vi "TonePattern-Initialize.vi"(0 "Tone Cloud":T2={"Freq"={"Min (Hz)"=500.0, "Max (Hz)"=8000.0, "#/octave"=4}, "Time"={"Duration (ms)"=50.0, "Interval (ms)"=50.0, "Ramp (ms)"=5.0}, "Pattern"={"# rand"=2.0, "reg fraction"=1.0, "Rcyc"=1, "pattern"=enum."REG", "Lsignal (cyc)"={"Min"=0, "Max"=0}, "Trans (cyc)"={"Min"=0, "Max"=0}}} caption="ToneCloud", 7 "Sampling rate (Hz)":dbl=50000.0, 9 "Npts":i32, 11 "error in (no error)":errorcluster) -> (3 "#frames":i32, 4 "Freqs":dbl[](array[numeric]), 8 "Data":T1={"Tones"=array2x2500[5000 elements], "Mask"=[1], "Index"=0, "pts/clock"=2500, "leftover"=0, "pts/tone"=0, "transition"=0, "nrepeat"=0}, 15 "error out":errorcluster)   [LabVIEW 2020]
uses:
  TonePattern-Properties.ctl
  TonePattern-Data.ctl
  TonePattern-Initialization Action.ctl
  Utility VIs/Math VIs/LinSpace (x0-dx-npts).vi
  Utility VIs/Array Manipulation VIs/Irregular Array Subset (I32).vi
  <vilib>/Analysis/1siggen.llb/Riffle Array (I32).vi
  <vilib>/Analysis/NI_AALBase.lvlib
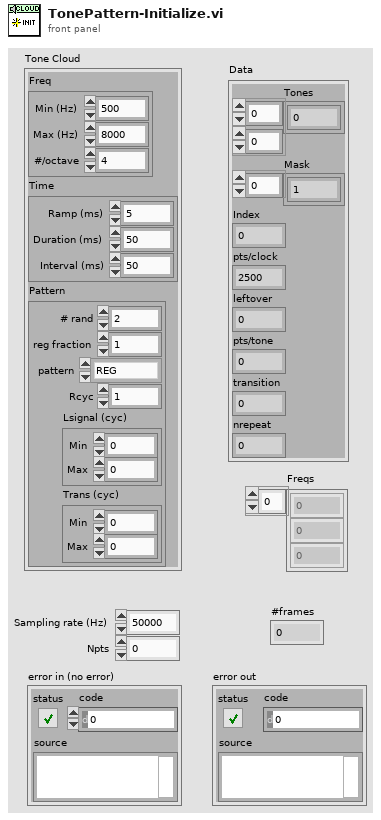
[diagram p1: front panel]
types:
  T1 = typedef "TonePattern-Data.ctl" = cluster{"Tones":dbl[][], "Mask":i32[], "Index":i32, "pts/clock":i32, "leftover":i32, "pts/tone":i32, "transition":i32, "nrepeat":i32}
  T2 = typedef "TonePattern-Properties.ctl" = cluster{"Freq":cluster{"Min (Hz)":dbl, "Max (Hz)":dbl, "#/octave":i32}, "Time":cluster{"Duration (ms)":dbl, "Interval (ms)":dbl, "Ramp (ms)":dbl}, "Pattern":cluster{"# rand":dbl, "reg fraction":dbl, "Rcyc":i32, "pattern":enum16{"RAND-REG", "REG-RAND", "RAND", "REG", "STEP", "CF"}, "Lsignal (cyc)":cluster{"Min":i32, "Max":i32}, "Trans (cyc)":cluster{"Min":i32, "Max":i32}}}
  T3 = typedef "TonePattern-Initialization Action.ctl" = enum16{"Tones", "Rand", "Reg", "Titrate", "Signal", "Done"}
  T4 = enum16{"RAND-REG", "REG-RAND", "RAND", "REG", "STEP", "CF"}
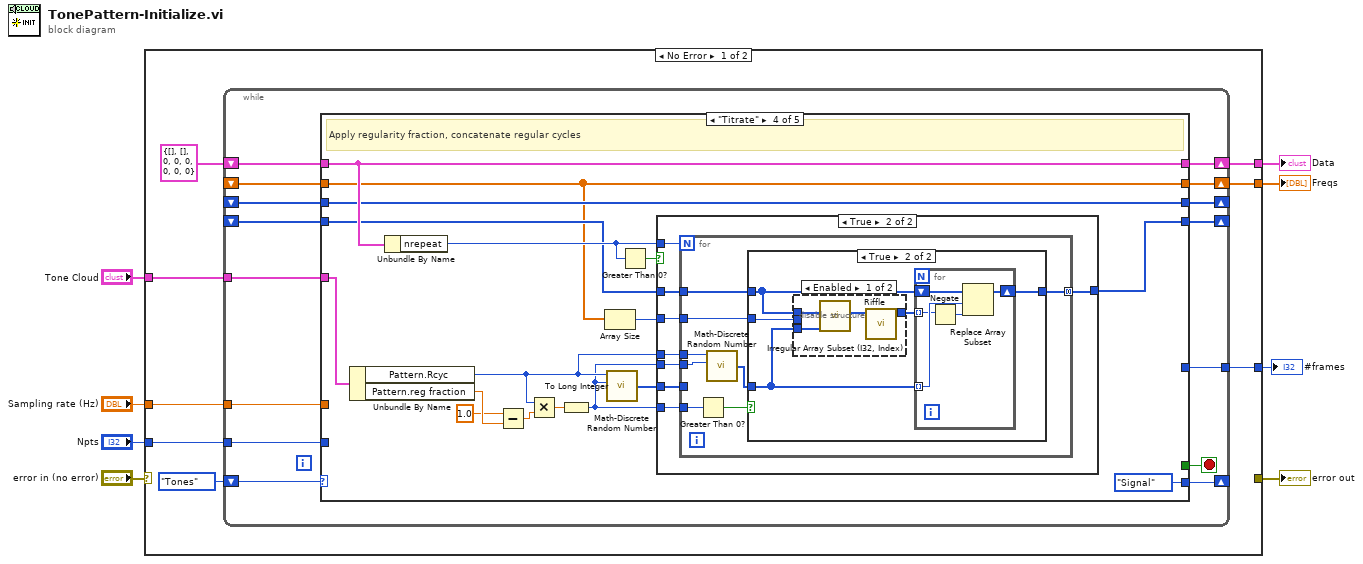
[diagram p0: block diagram]
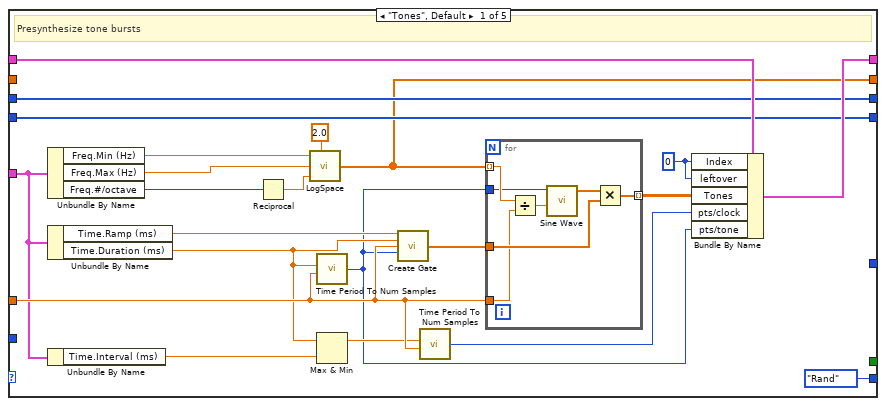
[diagram p2: hidden frame]
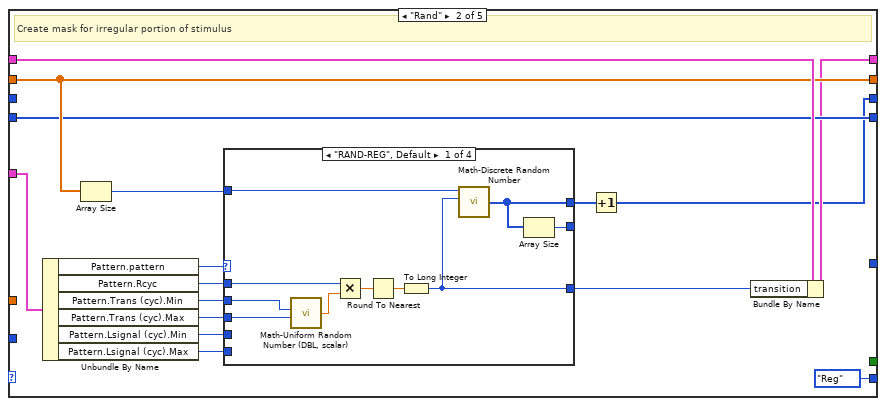
[diagram p3: hidden frame]
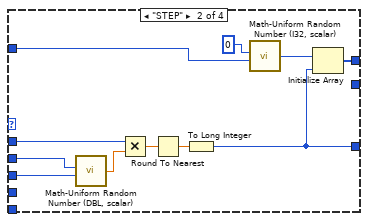
[diagram p4: hidden frame]
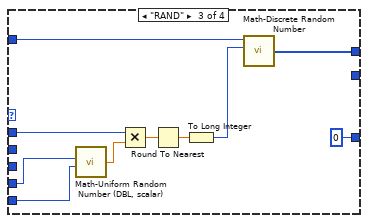
[diagram p5: hidden frame]
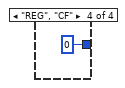
[diagram p6: hidden frame]
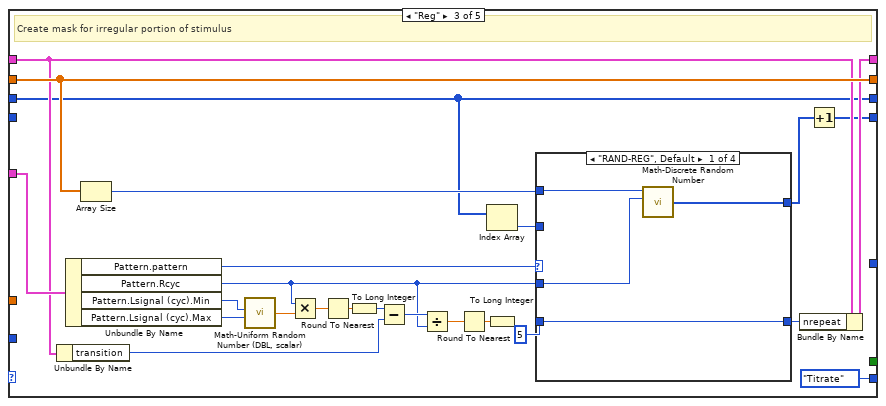
[diagram p7: hidden frame]
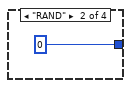
[diagram p8: hidden frame]
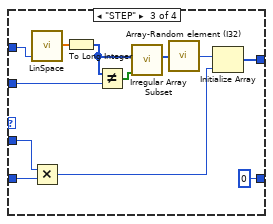
[diagram p9: hidden frame]
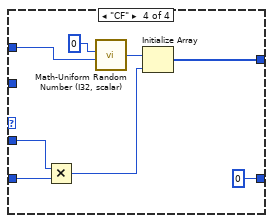
[diagram p10: hidden frame]
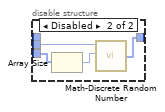
[diagram p13: hidden frame]
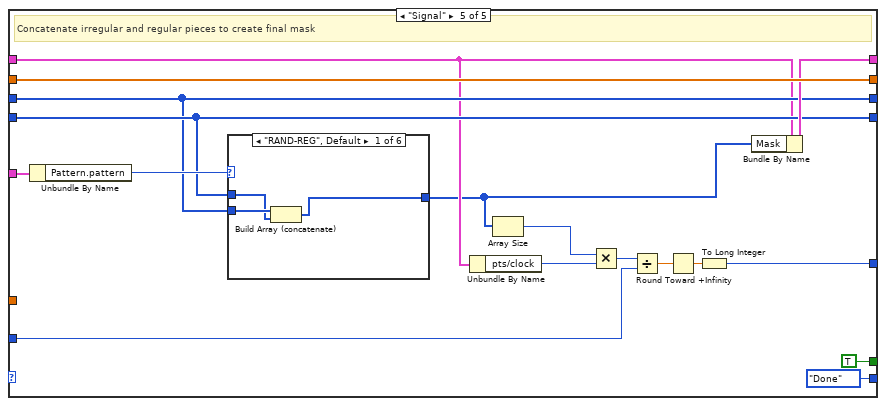
[diagram p14: hidden frame]
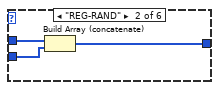
[diagram p15: hidden frame]
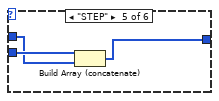
[diagram p18: hidden frame]
diagram:
  n1 = case shown="No Error" "error in (no error)" {
    selector: "error in (no error)" -> [_ w240]
    tunnel: [_ w240] -> w5
    tunnel: "Sampling rate (Hz)" -> [w15 _]
    tunnel: "Npts" -> [w11 _]
    tunnel: "Tone Cloud" -> [w14 _]
    tunnel: [w16 _] -> w3
    tunnel: [w12 _] -> w2
    tunnel: [w10 _] -> w1
    frame No Error {
      n2 = while {
        tunnel: w15 -> [w30]
        tunnel: w14 -> [w29]
        shift-right: [w31] -> w16
        shift-left: T1 {"Tones"=[], "Mask"=[], "Index"=0, "pts/clock"=0, "leftover"=0, "pts/tone"=0, "transition"=0, "nrepeat"=0} ("Data") -> [w28]
        shift-right: [w27] -> _
        shift-left: _ -> [w26]
        shift-right: [w25] -> w12
        shift-left: _ -> [w24]
        shift-right: [w23] -> _
        shift-left: _ -> [w22]
        tunnel: w11 -> [w20]
        tunnel: [w19] -> w10
        shift-right: [w17] -> _
        shift-left: TonePattern-Initialization_Action."Tones" -> [w18]
        stop <- w21 stop-if-true
        n3 = case shown="\"Titrate\"" w18 {
          tunnel: [w50 w66 w116 w173 w226] -> w31
          tunnel: w30 -> [w49 _ _ _ _]
          tunnel: w29 -> [w43 w76 w132 w172 w225]
          tunnel: w28 -> [w42 w75 w122 w173 w220]
          tunnel: [w41 w61 w112 w170 w222] -> w27
          tunnel: w26 -> [w41 _ w112 w170 w222]
          tunnel: [w35 w74 w131 w161 w227] -> w25
          tunnel: w24 -> [_ w74 w131 w161 w227]
          tunnel: [w40 w73 w109 w168 w223] -> w23
          tunnel: w22 -> [w40 w73 _ w162 w223]
          tunnel: [_ _ _ _ TRUE] -> w21
          tunnel: w20 -> [_ _ _ _ w215]
          tunnel: [_ _ _ _ w212] -> w19
          tunnel: [TonePattern-Initialization_Action."Rand" TonePattern-Initialization_Action."Reg" TonePattern-Initialization_Action."Titrate" TonePattern-Initialization_Action."Signal" TonePattern-Initialization_Action."Done"] -> w17
          frame "Tones", Default {
            w44 = 0 ("Index")
            # "Presynthesize tone bursts"
            n4 = Unbundle By Name(w43) -> ("Freq.Min (Hz)"=w34:dbl, "Freq.Max (Hz)"=w33:dbl, "Freq.#/octave"=w32:i32)
            n5 = Unbundle By Name(w43) -> ("Time.Ramp (ms)"=w53:dbl, "Time.Duration (ms)"=w47:dbl)
            n6 = Unbundle By Name(w43) -> ("Time.Interval (ms)"=w46:dbl)
            n7 = Reciprocal(x=w32) -> (1/x=w36:dbl)
            n8 = call "LogSpace.vi"("Start"=w34, "Base"=2.0, "Stop"=w33, "Step"=w36) -> ("Array"=w35:dbl[])  [unwired: 2 in, 1 out]
            n9 = call "Time Period To Num Samples.vi"("Duration (ms)"=w47, "Sampling rate (Hz)"=w49) -> ("Samples"=w39:i32)  [unwired: 5 in]
            n10 = Max & Min(x=w47, y=w46) -> (max(x,y)=w45:dbl)  [unwired: 1 out]
            n11 = call "Create Gate.vi"("Ramp (ms)"=w53, "Duration (ms)"=w47, "Sampling Rate (Hz)"=w49, "Npts"=w39) -> ("Gate"=w52:dbl[])  [unwired: 10 in, 1 out]
            n12 = call "Time Period To Num Samples.vi"("Duration (ms)"=w45, "Sampling rate (Hz)"=w49) -> ("Samples"=w48:i32)  [unwired: 5 in]
            n13 = for {
              tunnel: w35 -> [w58] mode=indexing
              tunnel: w52 -> [w60]
              tunnel: w39 -> [w55]
              tunnel: [w59] -> w51 mode=indexing
              tunnel: w49 -> [w57]
              n14 = Divide(x=w58, y=w57) -> (x/y=w56:dbl)
              n15 = call <vilib>:"Sine Wave.vi"("samples"=w55, "frequency"=w56) -> ("sine wave"=w54:dbl[])  [unwired: 3 in, 2 out]
              n16 = Multiply(x=w54, y=w60) -> (x*y=w59:dbl[])
            }
            n17 = Bundle By Name(cluster=w42, "Index"=w44, "leftover"=w44, "Tones"=w51, "pts/clock"=w48, "pts/tone"=w39) -> (w50:T1)
          }
          frame "Rand" {
            # "Create mask for irregular portion of stimulus"
            n18 = Unbundle By Name(w76) -> ("Pattern.pattern"=w64:T4, "Pattern.Rcyc"=w69:i32, "Pattern.Trans (cyc).Min"=w71:i32, "Pattern.Trans (cyc).Max"=w70:i32, "Pattern.Lsignal (cyc).Min"=w63:i32, "Pattern.Lsignal (cyc).Max"=w62:i32)
            n19 = Array Size(array=w74) -> (size(s)=w68:i32)
            n20 = case shown="\"RAND-REG\", Default" w64 {
              tunnel: w71 -> [w86 w97 _ _]
              tunnel: w70 -> [w85 w96 _ _]
              tunnel: w69 -> [w84 w95 w107 _]
              tunnel: w68 -> [w83 w91 w106 _]
              tunnel: [w78 w88 w105 _] -> w67
              tunnel: [w79 w87 0 0] -> w65
              tunnel: w63 -> [_ _ w100 _]
              tunnel: w62 -> [_ _ w99 _]
              tunnel: [w77 _ _ _] -> _
              frame "RAND-REG", Default {
                n21 = call "Math-Uniform Random Number (DBL, scalar).vi"("Ymax"=w85, "Ymin"=w86) -> ("Random Value"=w82:dbl)  [unwired: 4 in]
                n22 = Multiply(x=w84, y=w82) -> (x*y=w81:dbl)
                n23 = Round To Nearest(number=w81) -> (nearest integer value=w80:dbl)
                n24 = To Long Integer(number=w80) -> (32bit integer=w79:i32)
                n25 = call "Math-Discrete Random Number.vi"("N"=w79, "samples"=w83) -> ("Random Values"=w78:i32[])  [unwired: 4 in]
                n26 = Array Size(array=w78) -> (size(s)=w77:i32)
              }
              frame "STEP" {
                n27 = call "Math-Uniform Random Number (DBL, scalar).vi"("Ymax"=w96, "Ymin"=w97) -> ("Random Value"=w94:dbl)  [unwired: 4 in]
                n28 = Multiply(x=w95, y=w94) -> (x*y=w93:dbl)
                n29 = Round To Nearest(number=w93) -> (nearest integer value=w92:dbl)
                n30 = To Long Integer(number=w92) -> (32bit integer=w87:i32)
                n31 = call "Math-Uniform Random Number (I32, scalar).vi"("Ymax"=w91, "Ymin"=0) -> ("Random Int"=w89:i32)  [unwired: 4 in]
                n32 = Initialize Array(w89, w87) -> (w88:i32[])
              }
              frame "RAND" {
                n33 = call "Math-Uniform Random Number (DBL, scalar).vi"("Ymax"=w99, "Ymin"=w100) -> ("Random Value"=w104:dbl)  [unwired: 4 in]
                n34 = Multiply(x=w107, y=w104) -> (x*y=w103:dbl)
                n35 = Round To Nearest(number=w103) -> (nearest integer value=w102:dbl)
                n36 = To Long Integer(number=w102) -> (32bit integer=w101:i32)
                n37 = call "Math-Discrete Random Number.vi"("N"=w101, "samples"=w106) -> ("Random Values"=w105:i32[])  [unwired: 4 in]
              }
              frame "REG", "CF" {
              }
            }
            n38 = Increment(x=w67) -> (x+1=w61:i32[])
            n39 = Bundle By Name(cluster=w75, "transition"=w65) -> (w66:T1)
          }
          frame "Reg" {
            # "Create mask for irregular portion of stimulus"
            n40 = Unbundle By Name(w122) -> ("transition"=w120:i32)
            n41 = Unbundle By Name(w132) -> ("Pattern.pattern"=w114:T4, "Pattern.Rcyc"=w113:i32, "Pattern.Lsignal (cyc).Min"=w124:i32, "Pattern.Lsignal (cyc).Max"=w123:i32)
            n42 = Array Size(array=w131) -> (size(s)=w129:i32)
            n43 = call "Math-Uniform Random Number (DBL, scalar).vi"("Ymax"=w123, "Ymin"=w124) -> ("Random Value"=w125:dbl)  [unwired: 4 in]
            n44 = Multiply(x=w113, y=w125) -> (x*y=w126:dbl)
            n45 = Round To Nearest(number=w126) -> (nearest integer value=w127:dbl)
            n46 = To Long Integer(number=w127) -> (32bit integer=w121:i32)
            n47 = Subtract(x=w121, y=w120) -> (x-y=w119:i32)
            n48 = Divide(x=w119, y=w113) -> (x/y=w118:dbl)
            n49 = Round To Nearest(number=w118) -> (nearest integer value=w117:dbl)
            n50 = Index Array(array=w112) -> (element=w111:i32)  [unwired: 1 in]
            n51 = To Long Integer(number=w117) -> ()  [unwired: 1 out]
            n52 = case shown="\"RAND-REG\", Default" w114 {
              tunnel: w129 -> [w136 _ w142 w154]
              tunnel: [w135 _ w144 w150] -> w128
              tunnel: [w134 0 0 0] -> w115
              tunnel: 5 -> [w134 _ w147 w153]
              tunnel: w113 -> [w133 _ w146 w152]
              tunnel: w111 -> [_ _ w149 _]
              frame "RAND-REG", Default {
                n53 = call "Math-Discrete Random Number.vi"("N"=w133, "samples"=w136) -> ("Random Values"=w135:i32[])  [unwired: 4 in]
              }
              frame "RAND" {
              }
              frame "STEP" {
                n54 = call-poly "LinSpace.vi"("npts"=w142) -> ("Array"=w141:dbl[])  [unwired: 3 in, 1 out]
                n55 = Multiply(x=w146, y=w147) -> (x*y=w145:i32)
                n56 = To Long Integer(number=w141) -> (32bit integer=w139:i32[])
                n57 = Not Equal?(x=w139, y=w149) -> (x != y?=w140:bool[])
                n58 = call-poly "Irregular Array Subset.vi"("Mask"=w140, "Array"=w139) -> ("Array Subset"=w138:i32[])  [unwired: 8 in, 1 out]
                n59 = call "Array-Random element (I32).vi"("Array"=w138) -> ("Element"=w143:i32)  [unwired: 1 in, 1 out]
                n60 = Initialize Array(w143, w145) -> (w144:i32[])
              }
              frame "CF" {
                n61 = Multiply(x=w152, y=w153) -> (x*y=w151:i32)
                n62 = call "Math-Uniform Random Number (I32, scalar).vi"("Ymax"=w154, "Ymin"=0) -> ("Random Int"=w155:i32)  [unwired: 4 in]
                n63 = Initialize Array(w155, w151) -> (w150:i32[])
              }
            }
            n64 = Bundle By Name(cluster=w122, "nrepeat"=w115) -> (w116:T1)
            n65 = Increment(x=w128) -> (x+1=w109:i32[])
          }
          frame "Titrate" {
            # "Apply regularity fraction, concatenate regular cycles"
            n66 = Unbundle By Name(w172) -> ("Pattern.Rcyc"=w159:i32, "Pattern.reg fraction"=w164:dbl)
            n67 = Unbundle By Name(w173) -> ("nrepeat"=w167:i32)
            n68 = Subtract(x=1.0, y=w164) -> (x-y=w165:dbl)
            n69 = Multiply(x=w159, y=w165) -> (x*y=w171:dbl)
            n70 = To Long Integer(number=w171) -> (32bit integer=w158:i32)
            n71 = Array Size(array=w161) -> (size(s)=w160:i32)
            n72 = call "Math-Discrete Random Number.vi"("N"=w158, "samples"=w159) -> ("Random Values"=w169:i32[])  [unwired: 4 in]
            n73 = Greater Than 0?(x=w167) -> (x > 0?=w166:bool)
            n74 = case shown="True" w166 {
              tunnel: w167 -> [_ w183]
              tunnel: w162 -> [w175 w182]
              tunnel: w169 -> [_ w181]
              tunnel: w158 -> [_ w180]
              tunnel: [w175 w179] -> w168
              tunnel: w160 -> [_ w178]
              tunnel: w159 -> [_ w177]
              tunnel: w158 -> [_ w176]
              frame False {
              }
              frame True {
                n75 = for {
                  N: w183 -> [_]
                  tunnel: w182 -> [w189]
                  tunnel: w181 -> [_]
                  tunnel: w180 -> [w191]
                  tunnel: [w188] -> w179 mode=concatenating
                  tunnel: w178 -> [w187]
                  tunnel: w177 -> [w186]
                  tunnel: w176 -> [w185]
                  n76 = Greater Than 0?(x=w191) -> (x > 0?=w190:bool)
                  n77 = call "Math-Discrete Random Number.vi"("N"=w185, "samples"=w186) -> ("Random Values"=w184:i32[])  [unwired: 4 in]
                  n78 = case shown="True" w190 {
                    tunnel: w189 -> [w192 w197]
                    tunnel: w184 -> [_ w194]
                    tunnel: [w192 w196] -> w188
                    tunnel: w187 -> [_ w193]
                    frame False {
                    }
                    frame True {
                      n79 = disable-structure shown="Enabled" {
                        disable-tunnel: w197 -> [w200 _]
                        disable-tunnel: [w199 w202] -> w195
                        disable-tunnel: w194 -> [w198 w205]
                        disable-tunnel: w193 -> [_ w204]
                        frame Enabled {
                          n80 = call "Irregular Array Subset (I32, Index).vi"("Indices"=w198, "Array"=w200) -> ("Array Subset"=w201:i32[])  [unwired: 8 in, 1 out]
                          n81 = call-poly <vilib>:"Riffle.vi"("X"=w201) -> ("Riffled {X}"=w199:i32[])  [unwired: 8 in, 2 out]
                        }
                        frame Disabled {
                          n82 = Array Size(array=w205) -> (size(s)=w203:i32)
                          n83 = call "Math-Discrete Random Number.vi"("N"=w203, "samples"=w204) -> ("Random Values"=w202:i32[])  [unwired: 4 in]
                        }
                      }
                      n84 = for {
                        shift-right: [w209] -> w196
                        shift-left: w197 -> [w210]
                        tunnel: w195 -> [w207] mode=indexing
                        tunnel: w194 -> [w208] mode=indexing
                        n85 = Negate(x=w207) -> (-x=w206:i32)
                        n86 = Replace Array Subset(array=w210, new element=w206, index=w208) -> (w209:i32[])
                      }
                    }
                  }
                }
              }
            }
          }
          frame "Signal" {
            # "Concatenate irregular and regular pieces to create final mask"
            n87 = Unbundle By Name(w225) -> ("Pattern.pattern"=w224:T4)
            n88 = case shown="\"RAND-REG\", Default" w224 {
              tunnel: w223 -> [w229 w233 _ w235 w237 _]
              tunnel: w222 -> [w230 w232 w234 _ w238 w239]
              tunnel: [w228 w231 w234 w235 w236 w239] -> w219
              frame "RAND-REG", Default {
                n89 = Build Array (concatenate)(w230, w229) -> (w228:i32[])
              }
              frame "REG-RAND" {
                n90 = Build Array (concatenate)(w233, w232) -> (w231:i32[])
              }
              frame "RAND" {
              }
              frame "REG" {
              }
              frame "STEP" {
                n91 = Build Array (concatenate)(w238, w237) -> (w236:i32[])
              }
              frame "CF" {
              }
            }
            n92 = Unbundle By Name(w220) -> ("pts/clock"=w217:i32)
            n93 = Array Size(array=w219) -> (size(s)=w218:i32)
            n94 = Multiply(x=w218, y=w217) -> (x*y=w216:i32)
            n95 = Divide(x=w216, y=w215) -> (x/y=w214:dbl)
            n96 = Round Toward +Infinity(x=w214) -> (ceil(x): smallest int >= x=w213:dbl)
            n97 = To Long Integer(number=w213) -> (32bit integer=w212:i32)
            n98 = Bundle By Name(cluster=w220, "Mask"=w219) -> (w226:T1)
          }
        }
      }
    }
    frame Error {
    }
  }
  "error out" <- w5
  "Data" <- w3
  "Freqs" <- w2
  "#frames" <- w1
